vi "Check datatype.vi"(10 "Datatype":string[](array[string]), 11 "Data Array":string[][](array[string])) -> (3 "Array":T1(array[cluster]))   [LabVIEW 2020]
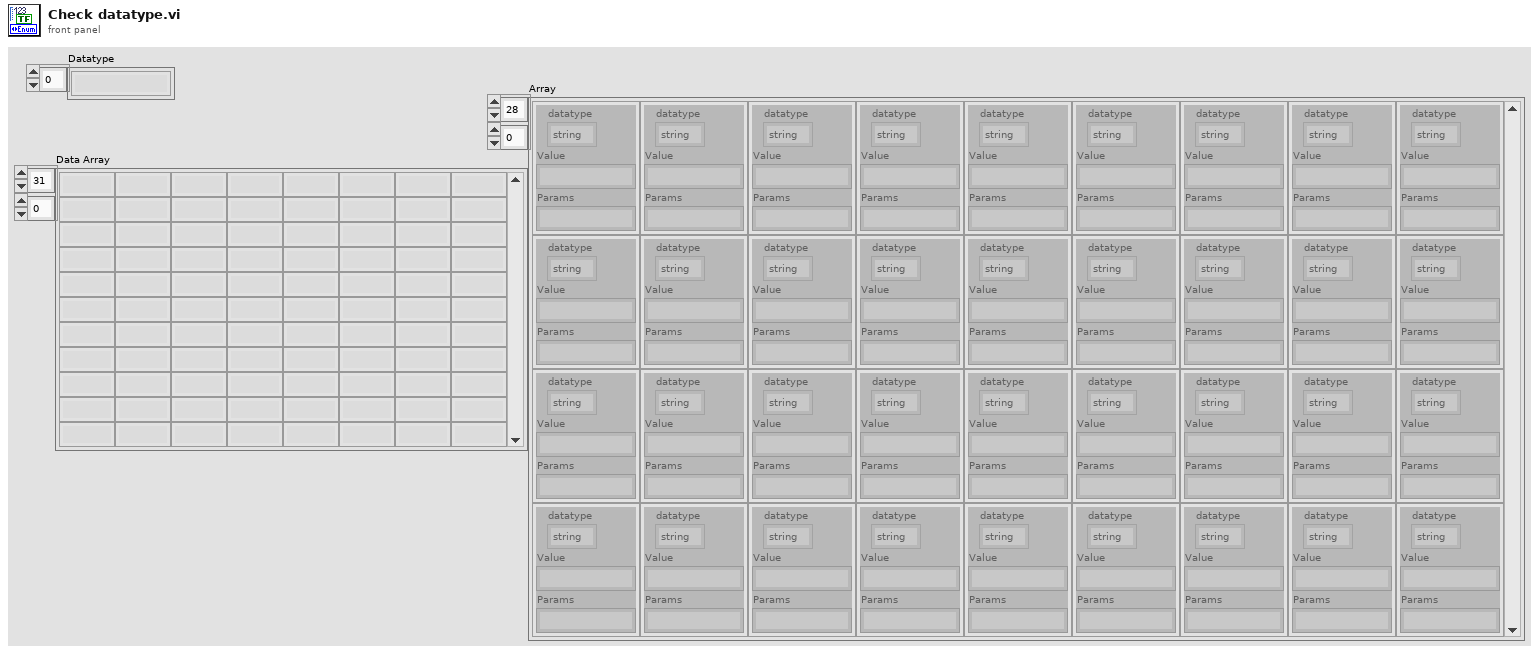
[diagram p1: front panel]
types:
  T1 = cluster{"datatype":enum16{"string", "image", "check", "numeric", "timestamp", "button", "combo", "link"}, "Value":string, "Params":string}[][]
  T2 = enum16{"string", "image", "check", "numeric", "timestamp", "button", "combo", "link"}
  T3 = cluster{"datatype":enum16{"string", "image", "check", "numeric", "timestamp", "button", "combo", "link"}, "Value":string, "Params":string}
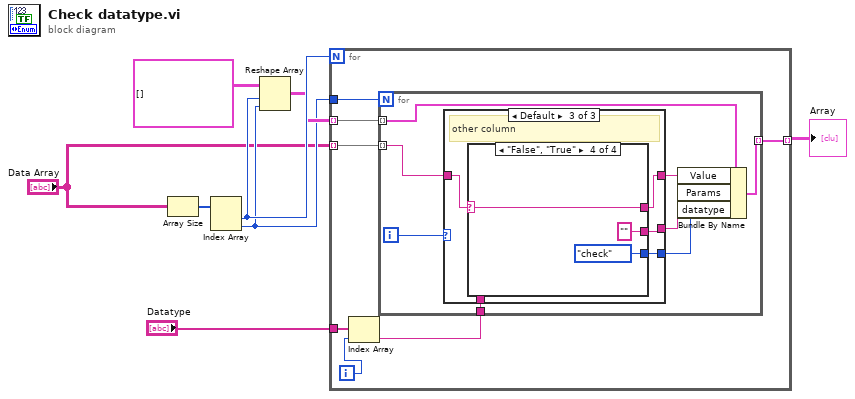
[diagram p0: block diagram]
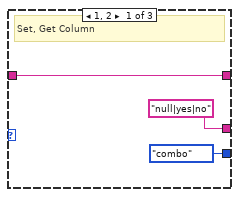
[diagram p2: hidden frame]
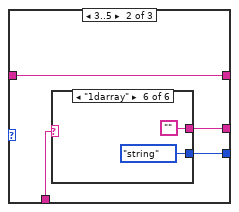
[diagram p3: hidden frame]
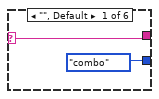
[diagram p4: hidden frame]
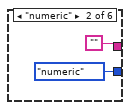
[diagram p5: hidden frame]
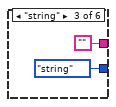
[diagram p6: hidden frame]
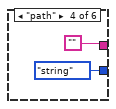
[diagram p7: hidden frame]
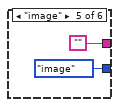
[diagram p8: hidden frame]
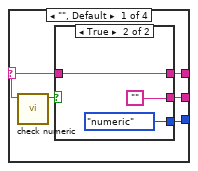
[diagram p9: hidden frame]
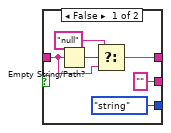
[diagram p10: hidden frame]
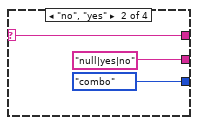
[diagram p11: hidden frame]
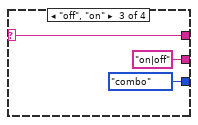
[diagram p12: hidden frame]
diagram:
  n1 = Array Size(array="Data Array") -> (size(s)=w3:i32[])
  n2 = Index Array(array=w3) -> (element #1=w8:i32, element #2=w6:i32)  [unwired: 2 in]
  n3 = Reshape Array(T1 [] ("Cells"), w8, w6) -> (w7:T1)
  n4 = for {
    N: w8 -> [_]
    tunnel: w6 -> [w15]
    tunnel: w7 -> [w14] mode=indexing
    tunnel: "Data Array" -> [w13] mode=indexing
    tunnel: [w12] -> w4 mode=indexing
    tunnel: "Datatype" -> [w11]
    i -> [w10]
    n5 = Index Array(array=w11, index=w10) -> (element=w9:string)
    n6 = for {
      N: w15 -> [_]
      tunnel: w14 -> [w23] mode=indexing
      tunnel: w13 -> [w21] mode=indexing
      tunnel: [w22] -> w12 mode=indexing
      tunnel: w9 -> [w16]
      i -> [w17]
      n7 = case shown="Default" w17 {
        tunnel: w21 -> [w26 w30 w46]
        tunnel: ["null|yes|no" w28 w45] -> w20
        tunnel: [T2."combo" ("datatype") w27 w44] -> w19
        tunnel: [w26 w30 w43] -> w18
        tunnel: w16 -> [_ w29 _]
        frame 1, 2 {
          # "Set, Get Column"
        }
        frame 3..5 {
          n8 = case shown="\"1darray\"" w29 {
            selector: w29 -> [w31 _ _ _ _ _]
            tunnel: [w31 "" "" "" "" ""] -> w28
            tunnel: [T2."combo" ("datatype") T2."numeric" ("datatype") T2."string" ("datatype") T2."string" ("datatype") T2."image" ("datatype") T2."string" ("datatype")] -> w27
            frame "", Default {
            }
            frame "numeric" {
            }
            frame "string" {
            }
            frame "path" {
            }
            frame "image" {
            }
            frame "1darray" {
            }
          }
        }
        frame Default {
          # "other column"
          n9 = case shown="\"False\", \"True\"" w46 {
            selector: w46 -> [w50 w61 w65 w69]
            tunnel: [w48 "null|yes|no" "on|off" ""] -> w45
            tunnel: [w47 T2."combo" ("datatype") T2."combo" ("datatype") T2."check" ("datatype")] -> w44
            tunnel: [w49 w61 w65 w69] -> w43
            frame "", Default {
              n10 = call "check numeric.vi"("String"=w50) -> ("all numeric?"=w51:bool)  [unwired: 10 in]
              n11 = case shown="True" w51 {
                tunnel: w50 -> [w54 w60]
                tunnel: [w52 w60] -> w49
                tunnel: ["" ""] -> w48
                tunnel: [T2."string" ("datatype") T2."numeric" ("datatype")] -> w47
                frame False {
                  n12 = Empty String/Path?(string/path=w54) -> (empty?=w55:bool)
                  n13 = Select(t="null", s=w55, f=w54) -> (s? t:f=w52:string)
                }
                frame True {
                }
              }
            }
            frame "no", "yes" {
            }
            frame "off", "on" {
            }
            frame "False", "True" {
            }
          }
        }
      }
      n14 = Bundle By Name(cluster=w23, "Value"=w18, "Params"=w20, "datatype"=w19) -> (w22:T3)
    }
  }
  "Array" <- w4
